vi "Status.vi"(8 "error in (no error)":errorcluster) -> (0 "error out":errorcluster, 1 "Status Explanation":string, 2 "Status as String":string, 3 "Status":T1)   [LabVIEW 2019, in "ACSVcontrol-driver.lvlib"]
doc: "Read status of the PJVS."
uses:
  ACSVcontrol-driver.lvlib
  Private/Type definitions/Status.ctl
  Private/Type definitions/Instruction.ctl
  Private/Globals.vi
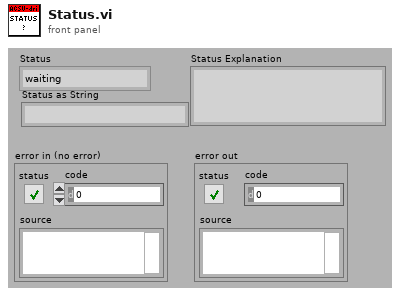
[diagram p1: front panel]
types:
  T1 = typedef "ACSVcontrol-driver.lvlib/Status.ctl" = enum16{"waiting", "processing", "error command", "Set_PJVS-Done", "Set_Mux-Done", "Set_Mux-Error", "Set_57XX-Done", "Set_57XX-Error", "Set_Gen-Done", "Set_Gen-Error", "Set_Synthesizer-Done", "Set_Synthesizer-Error", "Read_Nano-Done", "Read_Sampler-Done", "Read_Sampler-Error", "Read_Sensors-Done"}
  T2 = typedef "ACSVcontrol-driver.lvlib/Instruction.ctl" = enum16{"dummy - do not use", "Send Command", "Read Result", "Ask Status"}
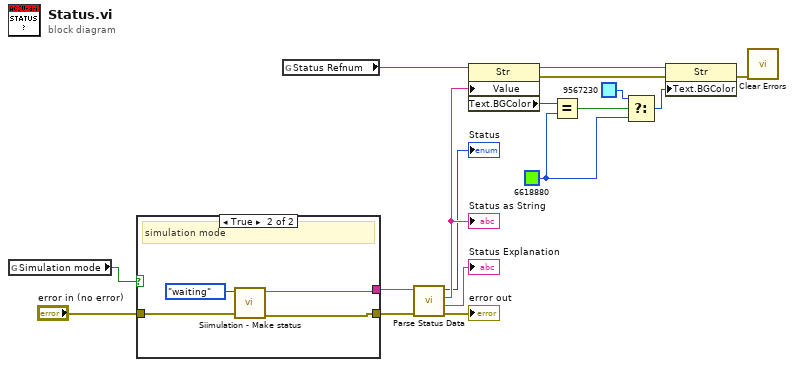
[diagram p0: block diagram]
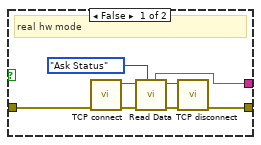
[diagram p2: hidden frame]
diagram:
  w6 = u32 6618880 ("Text.Text Colors:BG Color")
  n1 = global read "Globals.vi" "Simulation mode"() -> (w1:bool)
  n2 = case shown="True" w1 {
    tunnel: "error in (no error)" -> [w23 w29]
    tunnel: [w20 w26] -> w12
    tunnel: [w18 w28] -> w11
    frame False {
      # "real hw mode"
      n3 = call "TCP connect.vi"("error in (no error)"=w23) -> ("error out"=w22:errorcluster, "connection ID"=w24:refnum<k5>)  [unwired: 9 in]
      n4 = call "Read Data.vi"("Instruction"=Instruction."Ask Status", "error in (no error)"=w22, "connection ID"=w24) -> ("error out"=w19:errorcluster, "connection ID out"=w25:refnum<k5>, "Data"=w20:string)  [unwired: 6 in]
      n5 = call "TCP disconnect.vi"("error in (no error)"=w19, "connection ID"=w25) -> ("error out"=w18:errorcluster)  [unwired: 9 in]
    }
    frame True {
      # "simulation mode"
      n6 = call "Siimulation - Make status.vi"("error in (no error)"=w29, "Status"=Status."waiting") -> ("error out"=w28:errorcluster, "Status"=w26:string)  [unwired: 8 in]
    }
  }
  n7 = global read "Globals.vi" "Status Refnum"() -> (w13:refnum<vi>)
  n8 = call "Parse Status Data.vi"("error in"=w11, "Data"=w12) -> ("error out"=→"error out":errorcluster, "Status Explanation"=→"Status Explanation":string, "Status String"=w16:string, "Status"=→"Status":T1)  [unwired: 5 in, 1 out]
  "Status as String" <- w16
  n9 = property class="Str"(reference=w13, "Value"=w16) -> (reference out=w2:refnum<vi>, error out=w5:errorcluster, "Text.BGColor"=w9:u32)  [unwired: 1 in]
  n10 = Equal?(x=w9, y=w6) -> (x = y?=w8:bool)
  n11 = Select(t=u32 9567230 ("Text.Text Colors:BG Color"), s=w8, f=w6) -> (s? t:f=w3:u32)
  n12 = property class="Str"(reference=w2, error in=w5, "Text.BGColor"=w3) -> (error out=w4:errorcluster)  [unwired: 1 out]
  n13 = call <vilib>:"Clear Errors.vi"("error in (no error)"=w4) -> ()  [unwired: 5 in, 2 out]
